vi "Pair.vi"() -> ()   [LabVIEW 2025]
uses:
  libzmq-v143-mt-4_3_6/ctls/SocketType.ctl
  zeromq/Receive_string.vi
  zeromq/Send_string.vi
  zeromq/Context.lvclass
  libzmq-v143-mt-4_3_6/LibZMQ.lvlib
  zeromq/Socket.lvclass
panel:
  out "error out 3":errorcluster
  out "Routed back 3":string
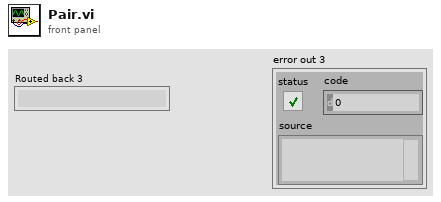
[diagram p1: front panel]
types:
  T1 = typedef "LibZMQ.lvlib/SocketType.ctl" = enum8{"PAIR", "PUB", "SUB", "REQ", "REP", "DEALER", "ROUTER", "PULL", "PUSH", "XPUB", "XSUB", "STREAM"}
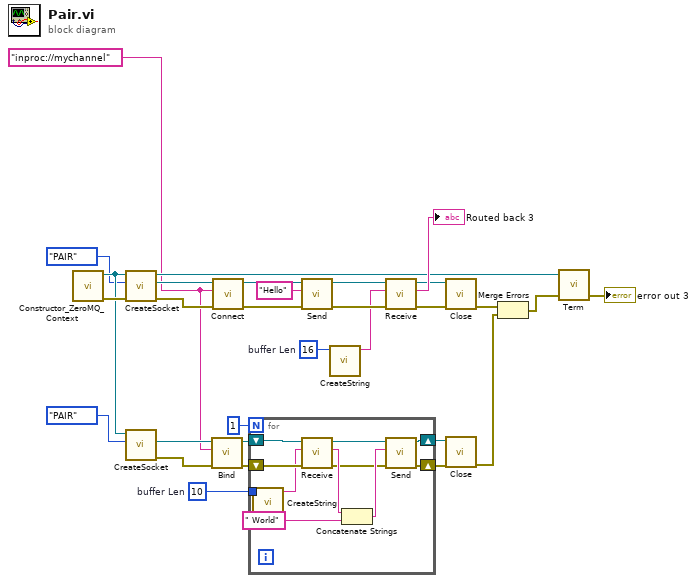
[diagram p0: block diagram]
diagram:
  w17 = 16  # buffer Len
  w23 = 10  # buffer Len
  w2 = "inproc://mychannel"
  n1 = call "Constructor_ZeroMQ_Context.vi"() -> ("error out"=w27:errorcluster, "context out"=w4:refnum<class "Context.lvclass">)  [unwired: 10 in]
  n2 = call "CreateSocket.vi"("error in"=w27, "Socket Type"=SocketType."PAIR", "context in"=w4) -> ("error out"=w12:errorcluster, "socket out"=w14:refnum<class "Socket.lvclass">, "context out"=w8:refnum<class "Context.lvclass">)  [unwired: 6 in]
  n3 = call "CreateSocket.vi"("Socket Type"=SocketType."PAIR", "context in"=w4) -> ("error out"=w24:errorcluster, "socket out"=w25:refnum<class "Socket.lvclass">)  [unwired: 7 in, 1 out]
  n4 = call "Bind.vi"("error in"=w24, "endpoint"=w2, "socket in"=w25) -> ("error out"=w21:errorcluster, "socket out"=w22:refnum<class "Socket.lvclass">)  [unwired: 7 in]
  n5 = call "Connect.vi"("error in"=w12, "endpoint"=w2, "socket in"=w14) -> ("error out"=w11:errorcluster, "socket out"=w13:refnum<class "Socket.lvclass">)  [unwired: 7 in]
  n6 = for {
    N: 1 -> [_]
    tunnel: w23 -> [w41]
    shift-right: [w32] -> w7
    shift-left: w22 -> [w40]
    shift-right: [w31] -> w6
    shift-left: w21 -> [w39]
    n7 = call "CreateString.vi"("length"=w41) -> ("string"=w38:string)  [unwired: 10 in]
    n8 = call-poly "Receive.vi"("error in"=w39, "buf in"=w38, "socket in"=w40) -> ("error out"=w33:errorcluster, "data"=w36:string, "socket out"=w37:refnum<class "Socket.lvclass">)  [unwired: 6 in]
    n9 = Concatenate Strings(w36, " World") -> (w34:string)
    n10 = call-poly "Send.vi"("error in"=w33, "data"=w34, "socket in"=w37) -> ("error out"=w31:errorcluster, "socket out"=w32:refnum<class "Socket.lvclass">)  [unwired: 7 in]
  }
  n11 = call-poly "Send.vi"("error in"=w11, "data"="Hello", "socket in"=w13) -> ("error out"=w18:errorcluster, "socket out"=w19:refnum<class "Socket.lvclass">)  [unwired: 7 in]
  n12 = call "CreateString.vi"("length"=w17) -> ("string"=w16:string)  [unwired: 10 in]
  n13 = call-poly "Receive.vi"("error in"=w18, "buf in"=w16, "socket in"=w19) -> ("error out"=w9:errorcluster, "data"=→"Routed back 3":string, "socket out"=w10:refnum<class "Socket.lvclass">)  [unwired: 6 in]
  n14 = call "Close.vi"("error in"=w9, "socket"=w10) -> ("error out"=w28:errorcluster)  [unwired: 9 in]
  n15 = call "Close.vi"("error in"=w6, "socket"=w7) -> ("error out"=w5:errorcluster)  [unwired: 9 in]
  n16 = Merge Errors(w28, w5) -> (w29:errorcluster)
  n17 = call "Term.vi"("error in"=w29, "context in"=w8) -> ("error out"=→"error out 3":errorcluster)  [unwired: 3 in]
